vi "StepTypetoStepClass.vi"(10 "StepTypeEnum":T1) -> (2 "AbstractStep out":refnum<class "AbstractStep.lvclass">)   [LabVIEW 2014, in "AbstractStep.lvclass"]
uses:
  AbstractStep.lvclass
  StepData/Control/StepTypeEnum.ctl
  Move/Move.lvclass
  Measure/Measure.lvclass
  StepData/StepData.lvclass
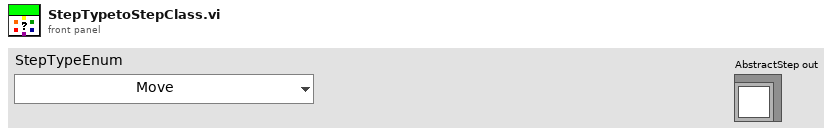
[diagram p1: front panel]
types:
  T1 = typedef "StepData.lvclass/StepTypeEnum.ctl" = enum16{"Move", "Measure"}
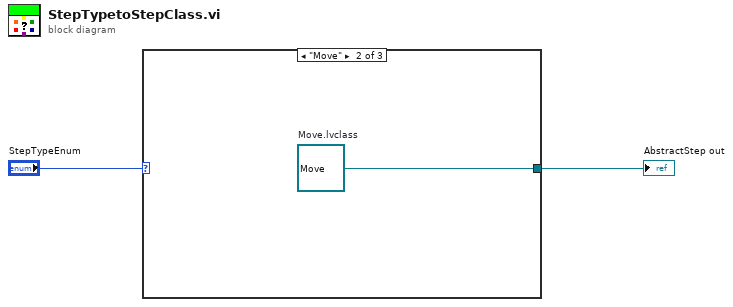
[diagram p0: block diagram]
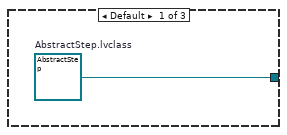
[diagram p2: hidden frame]
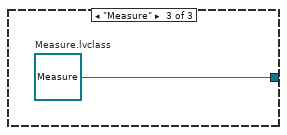
[diagram p3: hidden frame]
diagram:
  n1 = case shown="\"Move\"" "StepTypeEnum" {
    tunnel: [w3 w4 w5] -> w1
    frame Default {
      w3 = refnum<class "AbstractStep.lvclass"> refnum  # AbstractStep.lvclass
    }
    frame "Move" {
      w4 = refnum<class "Move.lvclass"> refnum  # Move.lvclass
    }
    frame "Measure" {
      w5 = refnum<class "Measure.lvclass"> refnum  # Measure.lvclass
    }
  }
  "AbstractStep out" <- w1
